vi "Write Loop Period in ms (10).vi"(8 "error in (no error)":errorcluster, 10 "Loop Period in ms (10)":u32=10, 11 "Analog Reader Helper in":refnum<class "Analog Reader Helper.lvclass">) -> (0 "error out":errorcluster, 3 "Analog Reader Helper out":refnum<class "Analog Reader Helper.lvclass">)   [LabVIEW 2024]
uses:
  Analog Reader Helper.lvclass
  Analog Reader Helper.lvclass/Analog Reader Helper.ctl
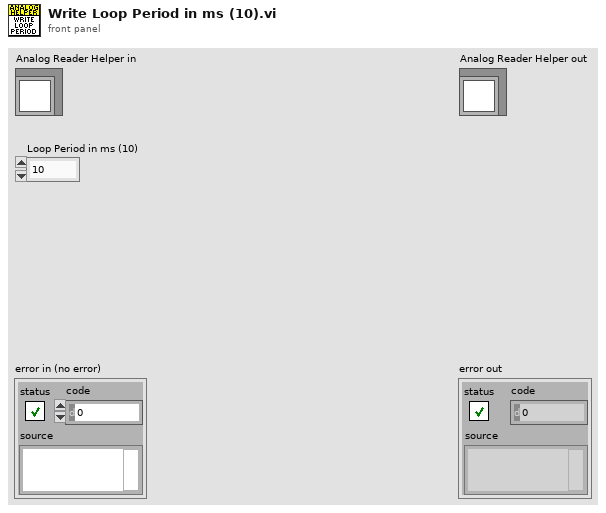
[diagram p1: front panel]
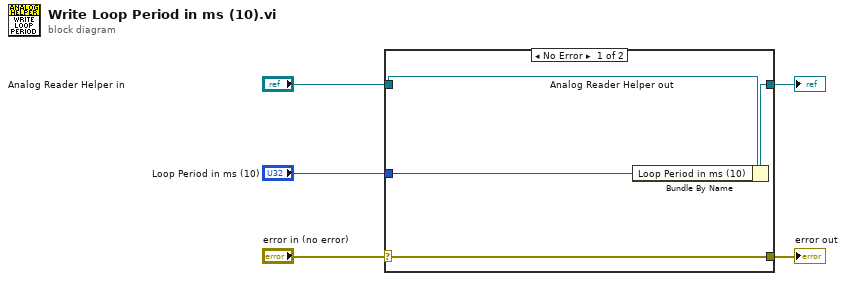
[diagram p0: block diagram]
diagram:
  n1 = case shown="No Error" "error in (no error)" {
    selector: "error in (no error)" -> [w9 w10]
    tunnel: [w9 w10] -> w4
    tunnel: [w7 w11] -> w2
    tunnel: "Analog Reader Helper in" -> [w8 w11]
    tunnel: "Loop Period in ms (10)" -> [w6 _]
    frame No Error {
      n2 = Bundle By Name(cluster=w8, "Loop Period in ms (10)"=w6) -> (w7:refnum<class "Analog Reader Helper.lvclass">)
    }
    frame Error {
    }
  }
  "error out" <- w4
  "Analog Reader Helper out" <- w2
